vi "PathPlanner_Constraints_New.vi"(8 "MaxAngularAccRadPSecSq":dbl, 9 "MaxAngularVelRadPsEc;":dbl, 10 "MaxAccelerationMpsSq;":dbl, 11 "MaxVelocityMps;":dbl) -> (3 "PathPlannerConstraints":T1)   [LabVIEW 2019, in "PathPlanner24.lvlib"]
doc: "/**\n * Create a new path constraints object\n *\n * @param maxVelocityMps Max linear velocity (M/S)\n * @param maxAccelerationMpsSq Max linear acceleration (M/S^2)\n * @param maxAngularVelocityRps Max angular velocity (Rad/S)\n * @param maxAngularAccelerationRpsSq Max angular acceleration (Rad/S^2)\n */"
uses:
  TypeDef/PathPlannerConstraints.ctl
  PathPlanner24.lvlib
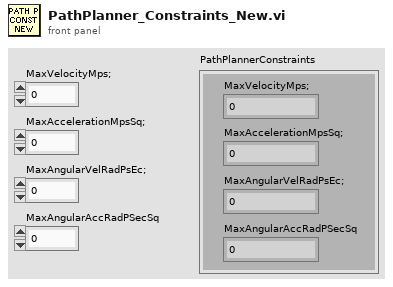
[diagram p1: front panel]
types:
  T1 = typedef "PathPlanner24.lvlib/PathPlannerConstraints.ctl" = cluster{"MaxVelocityMps;":dbl, "MaxAccelerationMpsSq;":dbl, "MaxAngularVelRadPsEc;":dbl, "MaxAngularAccRadPSecSq":dbl}
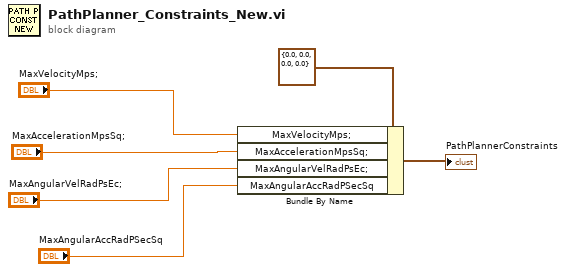
[diagram p0: block diagram]
diagram:
  n1 = Bundle By Name(cluster=T1 {"MaxVelocityMps;"=0.0, "MaxAccelerationMpsSq;"=0.0, "MaxAngularVelRadPsEc;"=0.0, "MaxAngularAccRadPSecSq"=0.0} ("PathPlannerConstraints"), "MaxVelocityMps;"="MaxVelocityMps;", "MaxAccelerationMpsSq;"="MaxAccelerationMpsSq;", "MaxAngularVelRadPsEc;"="MaxAngularVelRadPsEc;", "MaxAngularAccRadPSecSq"="MaxAngularAccRadPSecSq") -> (→"PathPlannerConstraints":T1)
